vi "Error if not an Agent.vi"(8 "error in (no error)":errorcluster, 11 "agent":T1) -> (0 "error out":errorcluster, 3 "agent out":T1)   [LabVIEW 2013, in "libssh2.lvlib"]
doc: "Reports an error if <B>agent</B> is not an agent."
uses:
  libssh2.lvlib
  Agent Refnum.ctl
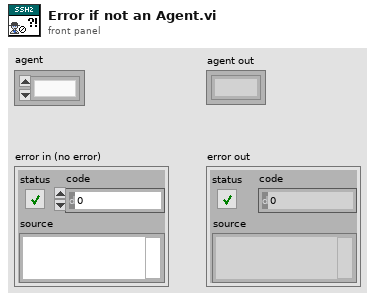
[diagram p1: front panel]
types:
  T1 = typedef "libssh2.lvlib/Agent Refnum.ctl" = refnum<k1>
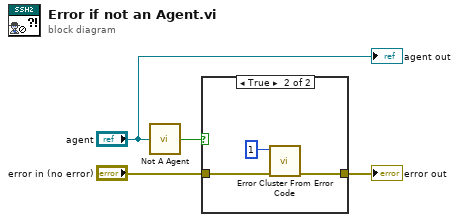
[diagram p0: block diagram]
diagram:
  n1 = call "Not A Agent.vi"("agent"="agent") -> ("Not a Agent?"=w2:bool)
  n2 = case shown="True" w2 {
    tunnel: "error in (no error)" -> [w5 w7]
    tunnel: [w5 w6] -> w3
    frame False {
    }
    frame True {
      n3 = call <vilib>:"Error Cluster From Error Code.vi"("error in (no error)"=w7, "error code (0)"=1) -> ("error out"=w6:errorcluster)  [unwired: 7 in]
    }
  }
  "error out" <- w3
  "agent out" <- "agent"
